vi "Recieve Request for Result.vi"(6 "Request time":timestamp, 8 "error in (no error)":errorcluster, 9 "Requestor":string, 10 "Requestee":string, 11 "Mag Lab Hardware in":refnum<class "Mag Lab Hardware.lvclass">) -> (0 "error out":errorcluster, 3 "Mag Lab Hardware out":refnum<class "Mag Lab Hardware.lvclass">)   [LabVIEW 2015, in "Mag Lab Hardware.lvclass"]
uses:
  Mag Lab Hardware.lvclass
  Mag Lab Root/Mag Lab Root.lvclass/Mag Lab Root.ctl
  Mag Lab Result/Mag Lab Result.lvclass/Mag Lab Result.ctl
  <vilib>/ActorFramework/Actor/Actor.lvclass/Actor.ctl
  Mag Lab Root Messages/Recieve Response with Result Msg/Recieve Response with Result Msg.lvclass/Recieve Response with Result Msg.ctl
  <vilib>/ActorFramework/Message Enqueuer/Message Enqueuer.lvclass/Message Enqueuer.ctl
  Mag Lab Result/Write Group Name.vi
  Mag Lab Result/Write Result time.vi
  <vilib>/ActorFramework/Message Enqueuer/Enqueue.vi
  <vilib>/ActorFramework/Message Priority Queue/Priority Enqueue.vi
  Mag Lab Root Messages/Recieve Response with Result Msg/Recieve Response with Result Msg.lvclass
  Mag Lab Root/Mag Lab Root.lvclass
  <vilib>/ActorFramework/Actor/Actor.lvclass
  Mag Lab Result/Mag Lab Result.lvclass
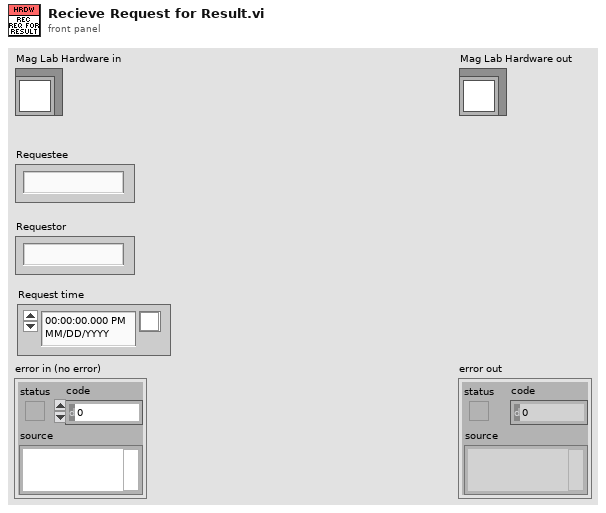
[diagram p1: front panel]
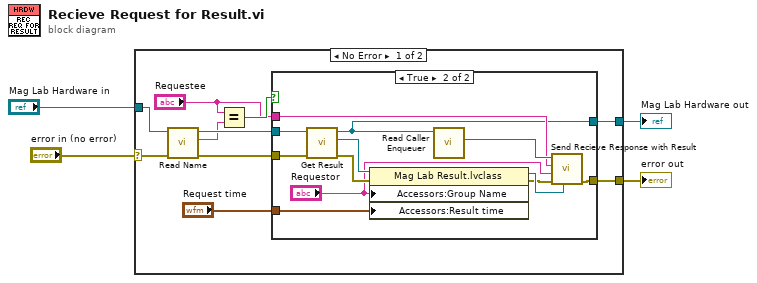
[diagram p0: block diagram]
diagram:
  n1 = case shown="No Error" "error in (no error)" {
    selector: "error in (no error)" -> [w11 w30]
    tunnel: [w14 w30] -> w3
    tunnel: [w13 w29] -> w1
    tunnel: "Mag Lab Hardware in" -> [w12 w29]
    frame No Error {
      n2 = call "Read Name.vi"("error in (no error)"=w11, "Mag Lab Root in"=w12) -> ("error out"=w8:errorcluster, "Name"=w6:string, "Mag Lab Root out"=w9:refnum<class "Mag Lab Hardware.lvclass">)  [unwired: 7 in]
      n3 = Equal?(x="Requestee", y=w6) -> (x = y?=w10:bool)
      n4 = case shown="True" w10 {
        tunnel: [w15 w25] -> w14
        tunnel: [w16 w24] -> w13
        tunnel: w9 -> [w16 w28]
        tunnel: "Requestee" -> [_ w26]
        tunnel: w8 -> [w15 w23]
        tunnel: "Request time" -> [_ w18]
        frame False {
        }
        frame True {
          n5 = call-dynamic "Get Result.vi"("error in (no error)"=w23, "Mag Lab Hardware in"=w28) -> ("error out"=w21:errorcluster, "Mag Lab Result.lvclass"=w19:refnum<class "Mag Lab Result.lvclass">, "Mag Lab Hardware out"=w24:refnum<class "Mag Lab Hardware.lvclass">)  [unwired: 7 in]
          n6 = property class="Mag Lab Result.lvclass"(reference=w19, error in=w21, "Accessors:Group Name"="Requestor", "Accessors:Result time"=w18) -> (reference out=w22:refnum<class "Mag Lab Result.lvclass">, error out=w20:errorcluster)
          n7 = call <vilib>:"Read Caller Enqueuer.vi"("Actor"=w24) -> ("Caller Enqueuer"=w27:refnum<class "Message Enqueuer.lvclass">)  [unwired: 10 in]
          n8 = call "Send Recieve Response with Result.vi"("Result"=w22, "error in (no error)"=w20, "Requestor"="Requestor", "Requestee"=w26, "Message Enqueuer"=w27) -> ("error out"=w25:errorcluster)  [unwired: 5 in, 1 out]
        }
      }
    }
    frame Error {
    }
  }
  "error out" <- w3
  "Mag Lab Hardware out" <- w1
